vi "Ballard - Arinc-429 RT Driver VI.vi"(7 "Operation":T1, 11 "Device Reference in":T2 format="%.0x") -> (0 "Error Code":i32)   [LabVIEW 2020, in "Ballard Arinc-429 Engine.lvlib"]
doc: "This VI is the Inline RT Driver VI."
uses:
  Ballard Arinc-429 Engine.lvlib
  <vilib>/NI VeriStand/Custom Device API/Custom Device Item Ref.ctl
  <vilib>/NI VeriStand/Custom Device API/Hardware Interface Driver VI Operation.ctl
  RT Controls/RT Asynchronous Parameters.ctl
  Shared/Controls and Global/RT HW Channel.ctl
  Shared/Controls and Global/RT Label Settings.ctl
  Shared/Controls and Global/Label.ctl
  Shared/Controls and Global/transferPeriod.ctl
  Shared/Controls and Global/RT Word Settings.ctl
  Shared/Controls and Global/RT Param Setting.ctl
  Shared/Controls and Global/Start Bit.ctl
  Shared/Controls and Global/Number of Bits.ctl
  <vilib>/NI VeriStand/Custom Device API/Block Data Reference.ctl
  <vilib>/NI VeriStand/Custom Device API/Data Reference.ctl
  Shared/Controls and Global/TransferType.ctl
  RT Controls/Tx_Maps.ctl
  RT Controls/RT Tx Association.ctl
  RT Controls/RT Tx Default Raw Value.ctl
  RT Controls/RT Tx Default Raw Value_Association.ctl
  RT Controls/RT Tx Association Trigger Channels.ctl
  RT Controls/RTStateVariables.ctl
  <vilib>/NI/NIVS Inline Async API/_VS Inline Async API/VS Inline Async API/VS Inline Async API.lvclass
  RT Controls/Card Parameters.ctl
  Shared/Controls and Global/Initialization Method.ctl
  RT Controls/Inline_Status_Channels.ctl
  <vilib>/NI/NIVS Inline Async API/_VS Inline Async API/VS Inline Async API/VS Inline Async API.lvclass/VS Inline Async API.ctl
  <vilib>/NI/NIVS Inline Async API/_Data Access Engine/Data Access Engine/Data Access Engine.lvclass/Data Access Engine.ctl
  <vilib>/NI/NIVS Inline Async API/_Data Access Engine/Access Type Classes/Write/Write.lvclass/Write.ctl
  <vilib>/NI/NIVS Inline Async API/_Data Access Engine/Access Type Classes/ReadWrite/ReadWrite.lvclass/ReadWrite.ctl
  <vilib>/NI/NIVS Inline Async API/_Data Access Engine/Access Type Classes/Read/Read.lvclass/Read.ctl
  <vilib>/NI/NIVS Inline Async API/_Data Access Engine/Data Access Engine/Methods/Data.Engine.Read Data from HW.vi
  <vilib>/NI/NIVS Inline Async API/_VS Inline Async API/Error Handling Process/SubVIs/Error.GetError.vi
  <vilib>/NI/NIVS Inline Async API/_Data Access Engine/Data Access Engine/Methods/Data.Engine.Write Data to HW.vi
  <vilib>/NI/NIVS Inline Async API/_Data Access Engine/Access Type Classes/ReadWrite/ReadWrite.EngineData.vi
  <vilib>/NI/NIVS Inline Async API/_Data Access Engine/Access Type Classes/Write/Write.EngineData.vi
  <vilib>/NI/NIVS Inline Async API/_Data Access Engine/Access Type Classes/Read/Read.EngineData.vi
  <vilib>/NI VeriStand/Custom Device API/NI VeriStand - Get Channel Value by Data Reference.vi
  <vilib>/NI VeriStand/Custom Device API/NI VeriStand - Set Channel Value by Data Reference.vi
  <vilib>/NI VeriStand/Custom Device API/NI VeriStand - Get Channel Values by Block Data Reference.vi
  <vilib>/NI VeriStand/Custom Device API/Global Data Refs.vi
  <vilib>/NI VeriStand/Custom Device Tools/Custom Device Utility Library/Custom Device Utility Library.lvlib
  Shared/Ballard Arinc-429 Shared.lvlib
  <vilib>/NI VeriStand/Custom Device API/Custom Device API.lvlib
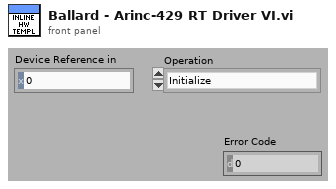
[diagram p1: front panel]
types:
  T1 = typedef "Custom Device API.lvlib/Hardware Interface Driver VI Operation.ctl" = enum16{"Initialize", "Start", "Read Data from HW", "Write Data to HW", "Close"}
  T2 = typedef "Custom Device API.lvlib/Custom Device Item Ref.ctl" = u64
  T3 = typedef "Ballard Arinc-429 Engine.lvlib/RTStateVariables.ctl" = cluster{"Async":refnum<class "VS Inline Async API.lvclass">, "Card Parameters (out)":T4, "Rx Config":T6[], "Inline Status Channels Refs":T15[]}
  T4 = typedef "Ballard Arinc-429 Engine.lvlib/Card Parameters.ctl" = cluster{"card number":i32, "core number":i32, "core handle":u64, "core reader handle":u64, "channel handles[]":u64[], "Initialization Method":T5, "PXI slot number":i32}
  T5 = typedef "Ballard Arinc-429 Shared.lvlib/Initialization Method.ctl" = enum16{"PXI Slot Number", "Card Number"}
  T6 = typedef "Ballard Arinc-429 Shared.lvlib/RT HW Channel.ctl" = cluster{"Labels Settings":T7[], "channel handle":u64, "channel #":u16}
  T7 = typedef "Ballard Arinc-429 Shared.lvlib/RT Label Settings.ctl" = cluster{"Name":string, "xmlName":string, "Label":T8, "transferPeriod":T9, "SDI_Enabled":bool, "SDI":u8, "Word":T10, "TransferType":T16, "has timestamp?":bool, "Label Disable/Trigger Channel Reference":T2, "Message Handle":u64, "Initialized?":bool, "Word Initial Raw Value":u32, "Label Timestamp Channel Data Reference":T15}
  T8 = typedef "Ballard Arinc-429 Shared.lvlib/Label.ctl" = u8
  T9 = typedef "Ballard Arinc-429 Shared.lvlib/transferPeriod.ctl" = u32
  T10 = typedef "Ballard Arinc-429 Shared.lvlib/RT Word Settings.ctl" = cluster{"Param Setting":T11}
  T11 = typedef "Ballard Arinc-429 Shared.lvlib/RT Param Setting.ctl" = cluster{"Start Bit":T12[], "Num Bits":T13[], "Signed?":bool[], "ScaleFac":dbl[], "ScaleOffset":dbl[], "Block Data Refs":T14[], "Encoding":enum16{"BNR", "BCD", "Discrete"}[], "Values Array":dbl[], "Item Refs":T2[]}
  T12 = typedef "Ballard Arinc-429 Shared.lvlib/Start Bit.ctl" = i32
  T13 = typedef "Ballard Arinc-429 Shared.lvlib/Number of Bits.ctl" = i32
  T14 = typedef "Custom Device API.lvlib/Block Data Reference.ctl" = cluster{"Data Reference":T15, "Offset":u64, "Length":u64}
  T15 = typedef "Custom Device API.lvlib/Data Reference.ctl" = i32
  T16 = typedef "Ballard Arinc-429 Shared.lvlib/TransferType.ctl" = enum16{"ScheduledLabel", "Acyclic", "Block", "Strobe"}
  T17 = typedef "Ballard Arinc-429 Engine.lvlib/RT Asynchronous Parameters.ctl" = cluster{"Input Channel Data []":T6[], "Maps":T18, "core handle":u64}
  T18 = typedef "Ballard Arinc-429 Engine.lvlib/Tx_Maps.ctl" = cluster{"Tx Map - Disable Channels":T19[], "Tx Map - Cyclic Labels - Parameters Channels":T19[], "Cyclic Labels - Raw Values":T20, "Tx Map - Trigger Channels":T22[], "Acyclic Labels - Raw Values":T20, "Tx Map - Acyclic Labels - Parameters Channels":T19[]}
  T19 = typedef "Ballard Arinc-429 Engine.lvlib/RT Tx Association.ctl" = cluster{"Channel Data Reference":T15, "Channel Index":i32, "Label Index":i32, "Parameter Index":i32, "Message Handle":u64, "Type":enum16{"Parameter Channel", "Disable/Trigger Channel"}}
  T20 = typedef "Ballard Arinc-429 Engine.lvlib/RT Tx Default Raw Value.ctl" = cluster{"Association":T21[], "Raw Values Array":u32[]}
  T21 = typedef "Ballard Arinc-429 Engine.lvlib/RT Tx Default Raw Value_Association.ctl" = cluster{"Channel Data Reference":T15, "Raw Value Index":i32}
  T22 = typedef "Ballard Arinc-429 Engine.lvlib/RT Tx Association Trigger Channels.ctl" = cluster{"Channel Data Reference":T15, "Channel Index":i32, "Label Index":i32, "Raw Value Index":i32, "channel handle":u64, "Type":enum16{"Parameter Channel", "Disable/Trigger Channel"}}
  T23 = typedef "Ballard Arinc-429 Engine.lvlib/Inline_Status_Channels.ctl" = enum16{"Error Code", "Inline Read Time (us)", "Inline Write Time (us)", "Receiving Error - Error Counter", "Gap Error - Error Counter", "Parity Error - Error Counter", "Long Word Error - Error Counter", "Bit Timing Error - Error Counter"}
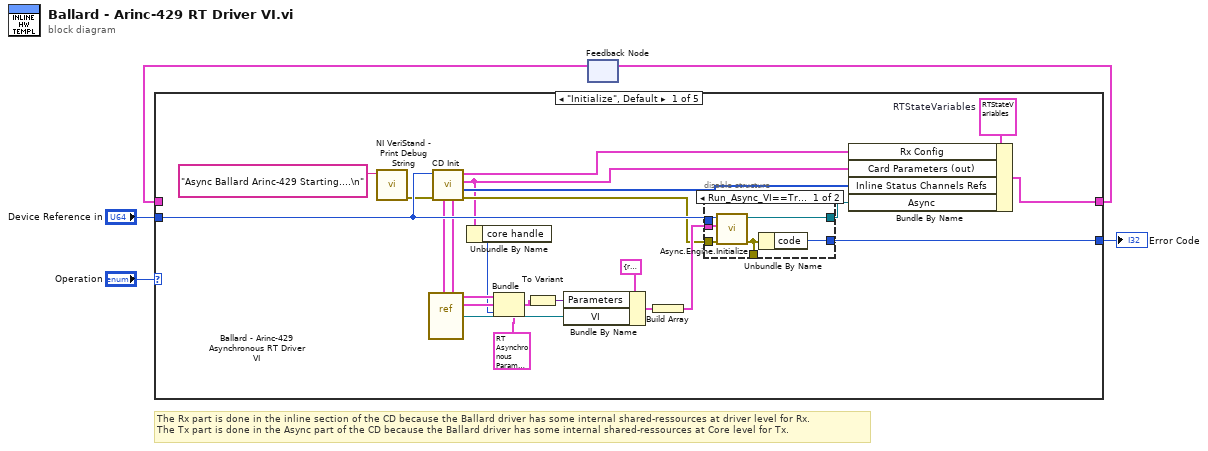
[diagram p0: block diagram]
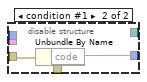
[diagram p2: hidden frame]
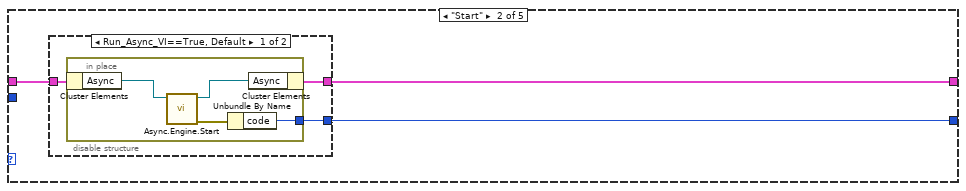
[diagram p3: hidden frame]
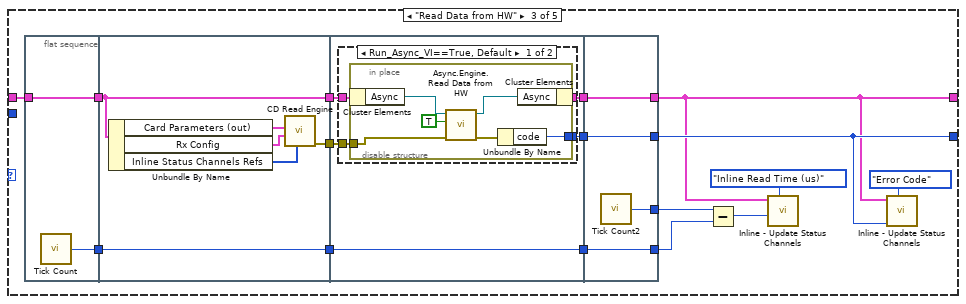
[diagram p5: hidden frame]
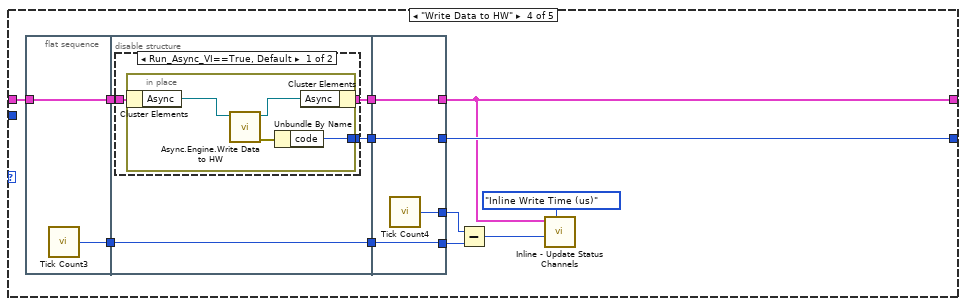
[diagram p7: hidden frame]
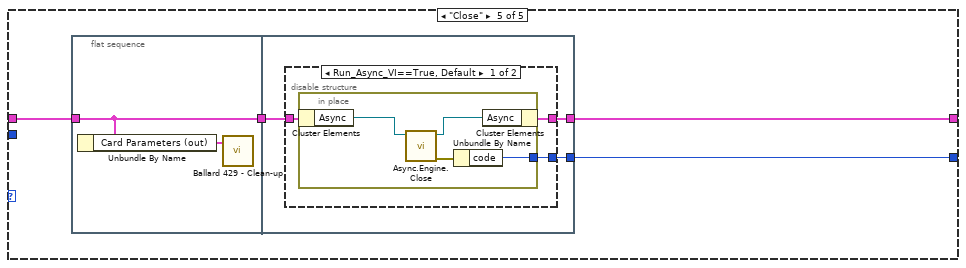
[diagram p9: hidden frame]
diagram:
  # "The Rx part is done in the inline section of the CD because the Ballard driver has some internal shared-ressources at driver level for Rx.\nThe Tx part is done in the Async part of the CD because the Ballard driver has some internal shared-ressources at Core level for Tx."
  n1 = feedback #1() -> (w3:T3)  [unwired: 1 out]
  n2 = case shown="\"Initialize\", Default" "Operation" {
    tunnel: [w24 w36 w52 w90 w122] -> w4
    tunnel: w3 -> [_ w37 w61 w100 w123]
    tunnel: "Device Reference in" -> [w17 _ _ _ _]
    tunnel: [w26 w35 w56 w101 w121] -> w1
    frame "Initialize", Default {
      w21 = T3 {"Async"=refnum, "Card Parameters (out)"={"card number"=0, "core number"=0, "core handle"=0, "core reader handle"=0, "channel handles[]"=[], "Initialization Method"=enum."PXI Slot Number", "PXI slot number"=0}, "Rx Config"=[], "Inline Status Channels Refs"=[]}  # RTStateVariables
      n3 = call <vilib>:"NI VeriStand - Print Debug String.vi"("Message"="Async Ballard Arinc-429 Starting....\n") -> ("error out"=w13:errorcluster)  [unwired: 10 in]
      n4 = vi-ref "Ballard - Arinc-429 Asynchronous RT Driver VI.vi"() -> (w18:refnum<vi>)
      n5 = call "CD Init.vi"("Error (in)"=w13, "Device Reference"=w17) -> ("Error (out)"=w14:errorcluster, "Inline Status Channels Refs"=w15:T15[], "Card Parameters (out)"=w7:T4, "Output Channel Data []"=w16:T6[], "Input Channel Data []"=w12:T6[], "Maps"=w11:T18)  [unwired: 4 in]
      n6 = Unbundle By Name(w7) -> ("core handle"=w6:u64)
      n7 = Bundle(cluster=T17 {"Input Channel Data []"=[], "Maps"={"Tx Map - Disable Channels"=[], "Tx Map - Cyclic Labels - Parameters Channels"=[], "Cyclic Labels - Raw Values"={"Association"=[], "Raw Values Array"=[]}, "Tx Map - Trigger Channels"=[], "Acyclic Labels - Raw Values"={"Association"=[], "Raw Values Array"=[]}, "Tx Map - Acyclic Labels - Parameters Channels"=[]}, "core handle"=0}, "Input Channel Data []"=w12, "Maps"=w11, "core handle"=w6) -> (w10:T17)
      n8 = To Variant(anything=w10) -> (Variant=w9:variant)
      n9 = Bundle By Name(cluster=cluster{"VI":refnum<vi>, "Parameters":variant} {"VI"=refnum, "Parameters"=variant} ("Process"), "Parameters"=w9, "VI"=w18) -> (w22:cluster{"VI":refnum<vi>, "Parameters":variant})
      n10 = Build Array(w22) -> (w20:cluster{"VI":refnum<vi>, "Parameters":variant}[])
      n11 = disable-structure shown="Run_Async_VI==True, Default" {
        disable-tunnel: [w32 w33] -> w26
        disable-tunnel: [w31 _] -> w25
        disable-tunnel: w20 -> [w30 _]
        disable-tunnel: w14 -> [w29 w34]
        disable-tunnel: w17 -> [w28 _]
        disable-tunnel: [w27 _] -> _
        frame condition #0 (active) {
          n12 = call <vilib>:"Async.Engine.Initialize.vi"("error in (no error)"=w29, "Processes"=w30, "Custom Device Ref"=w28) -> ("error out"=w27:errorcluster, "Async"=w31:refnum<class "VS Inline Async API.lvclass">)  [unwired: 7 in]
          n13 = Unbundle By Name(w27) -> ("code"=w32:i32)
        }
        frame condition #1 {
          n14 = Unbundle By Name(w34) -> ("code"=w33:i32)
        }
      }
      n15 = Bundle By Name(cluster=w21, "Rx Config"=w16, "Card Parameters (out)"=w7, "Inline Status Channels Refs"=w15, "Async"=w25) -> (w24:T3)
    }
    frame "Start" {
      n16 = disable-structure shown="Run_Async_VI==True, Default" {
        disable-tunnel: w37 -> [w40 w45]
        disable-tunnel: [w39 w45] -> w36
        disable-tunnel: [w38 _] -> w35
        frame condition #0 (active) {
          n17 = in-place {
            in-place-border: [w41] -> w38
            n18 = in-place-cluster #2(w40) -> ("Async"=w44:refnum<class "VS Inline Async API.lvclass">)
            n19 = call <vilib>:"Async.Engine.Start.vi"("VS Inline Async API in"=w44) -> ("error out"=w42:errorcluster, "VS Inline Async API out"=w43:refnum<class "VS Inline Async API.lvclass">)  [unwired: 9 in]
            n20 = Unbundle By Name(w42) -> ("code"=w41:i32)
            n21 = in-place-cluster #2("Async"=w43) -> (w39:T3)
          }
        }
        frame condition #1 {
        }
      }
    }
    frame "Read Data from HW" {
      n22 = flat-sequence {
        tunnel: w61 -> [w63]
        tunnel: [w63] -> w60
        tunnel: [w62] -> w59
        tunnel: [w68] -> w51
        tunnel: [w69] -> w49
        tunnel: w59 -> [w69]
        tunnel: w60 -> [w68]
        tunnel: [w67] -> w46
        tunnel: w51 -> [w72]
        tunnel: [w71] -> w50
        tunnel: w49 -> [w74]
        tunnel: [w74] -> w48
        tunnel: [w73] -> w47
        tunnel: w46 -> [w70]
        tunnel: [w88] -> w52
        tunnel: [w89] -> w56
        tunnel: w50 -> [w88]
        tunnel: [w87] -> w58
        tunnel: w48 -> [w86]
        tunnel: [w86] -> w57
        tunnel: w47 -> [w89]
        frame #0 {
          n23 = call "Tick Count"() -> ("Tick Count(uSec)"=w62:u32)
        }
        frame #1 {
          n24 = Unbundle By Name(w68) -> ("Card Parameters (out)"=w66:T4, "Rx Config"=w65:T6[], "Inline Status Channels Refs"=w64:T15[])
          n25 = call "CD Read Engine.vi"("Inline Status Channels Refs"=w64, "Output Channel Data []"=w65, "Card Parameters (in)"=w66) -> ("Error (out)"=w67:errorcluster)  [unwired: 7 in]
        }
        frame #2 {
          n26 = disable-structure shown="Run_Async_VI==True, Default" {
            disable-tunnel: [w78 _] -> w73
            disable-tunnel: w72 -> [w77 w85]
            disable-tunnel: [w76 w85] -> w71
            disable-tunnel: w70 -> [w75 _]
            frame condition #0 (active) {
              n27 = in-place {
                in-place-border: [w82] -> w78
                in-place-border: w75 -> [w79]
                n28 = in-place-cluster #3(w77) -> ("Async"=w84:refnum<class "VS Inline Async API.lvclass">)
                n29 = call <vilib>:"Async.Engine.Read Data from HW.vi"("error in"=w79, "Report Error to Inline?"=TRUE, "Async in"=w84) -> ("error out"=w81:errorcluster, "Async out"=w83:refnum<class "VS Inline Async API.lvclass">)  [unwired: 7 in]
                n30 = Unbundle By Name(w81) -> ("code"=w82:i32)
                n31 = in-place-cluster #3("Async"=w83) -> (w76:T3)
              }
            }
            frame condition #1 {
            }
          }
        }
        frame #3 {
          n32 = call "Tick Count2"() -> ("Tick Count(uSec)"=w87:u32)
        }
      }
      n33 = Subtract(x=w58, y=w57) -> (x-y=w53:u32)
      n34 = call "Inline - Update Status Channels.vi"("Status Channel"=Inline_Status_Channels."Inline Read Time (us)", "Time (us)"=w53, "RTStateVariables"=w52) -> ()  [unwired: 9 in]
      n35 = call "Inline - Update Status Channels.vi"("Status Channel"=Inline_Status_Channels."Error Code", "Error Code"=w56, "RTStateVariables"=w52) -> ()  [unwired: 9 in]
    }
    frame "Write Data to HW" {
      n36 = flat-sequence {
        tunnel: w100 -> [w103]
        tunnel: [w103] -> w99
        tunnel: [w102] -> w96
        tunnel: w99 -> [w104]
        tunnel: [w107] -> w98
        tunnel: [w106] -> w97
        tunnel: w96 -> [w105]
        tunnel: [w105] -> w95
        tunnel: [w118] -> w90
        tunnel: [w119] -> w101
        tunnel: w98 -> [w119]
        tunnel: w97 -> [w118]
        tunnel: [w117] -> w93
        tunnel: w95 -> [w116]
        tunnel: [w116] -> w94
        frame #0 {
          n37 = call "Tick Count3"() -> ("Tick Count(uSec)"=w102:u32)
        }
        frame #1 {
          n38 = disable-structure shown="Run_Async_VI==True, Default" {
            disable-tunnel: [w110 _] -> w107
            disable-tunnel: w104 -> [w109 w115]
            disable-tunnel: [w108 w115] -> w106
            frame condition #0 (active) {
              n39 = in-place {
                in-place-border: [w114] -> w110
                n40 = in-place-cluster #4(w109) -> ("Async"=w112:refnum<class "VS Inline Async API.lvclass">)
                n41 = call <vilib>:"Async.Engine.Write Data to HW.vi"("VS Inline Async API in"=w112) -> ("error out"=w113:errorcluster, "VS Inline Async API out"=w111:refnum<class "VS Inline Async API.lvclass">)  [unwired: 9 in]
                n42 = Unbundle By Name(w113) -> ("code"=w114:i32)
                n43 = in-place-cluster #4("Async"=w111) -> (w108:T3)
              }
            }
            frame condition #1 {
            }
          }
        }
        frame #2 {
          n44 = call "Tick Count4"() -> ("Tick Count(uSec)"=w117:u32)
        }
      }
      n45 = Subtract(x=w93, y=w94) -> (x-y=w91:u32)
      n46 = call "Inline - Update Status Channels.vi"("Status Channel"=Inline_Status_Channels."Inline Write Time (us)", "Time (us)"=w91, "RTStateVariables"=w90) -> ()  [unwired: 9 in]
    }
    frame "Close" {
      n47 = flat-sequence {
        tunnel: w123 -> [w125]
        tunnel: [w125] -> w120
        tunnel: [w127] -> w122
        tunnel: [w126] -> w121
        tunnel: w120 -> [w128]
        frame #0 {
          n48 = Unbundle By Name(w125) -> ("Card Parameters (out)"=w124:T4)
          n49 = call "Ballard 429 - Clean-up.vi"("Card Parameters (in)"=w124) -> ()  [unwired: 10 in, 1 out]
        }
        frame #1 {
          n50 = disable-structure shown="Run_Async_VI==True, Default" {
            disable-tunnel: w128 -> [w131 w136]
            disable-tunnel: [w130 w136] -> w127
            disable-tunnel: [w129 _] -> w126
            frame condition #0 (active) {
              n51 = in-place {
                in-place-border: [w133] -> w129
                n52 = in-place-cluster #5(w131) -> ("Async"=w135:refnum<class "VS Inline Async API.lvclass">)
                n53 = call <vilib>:"Async.Engine.Close.vi"("Async in"=w135) -> ("error out"=w132:errorcluster, "Async out"=w134:refnum<class "VS Inline Async API.lvclass">)  [unwired: 9 in]
                n54 = Unbundle By Name(w132) -> ("code"=w133:i32)
                n55 = in-place-cluster #5("Async"=w134) -> (w130:T3)
              }
            }
            frame condition #1 {
            }
          }
        }
      }
    }
  }
  "Error Code" <- w1
  n56 = feedback-in #1(w4) -> ()
